vi "Add Mux.vi"(8 "error in (no error)":errorcluster, 11 "Node Ptr":u64 format="%.0x") -> (0 "error out":errorcluster)   [LabVIEW 2013, in "MUX Custom Device.lvlib"]
uses:
  MUX Custom Device.lvlib
  MUX Global.vi
  <vilib>/NI Veristand/Custom Device API/Custom Device API.lvlib
panel:
  in  "Tag":string
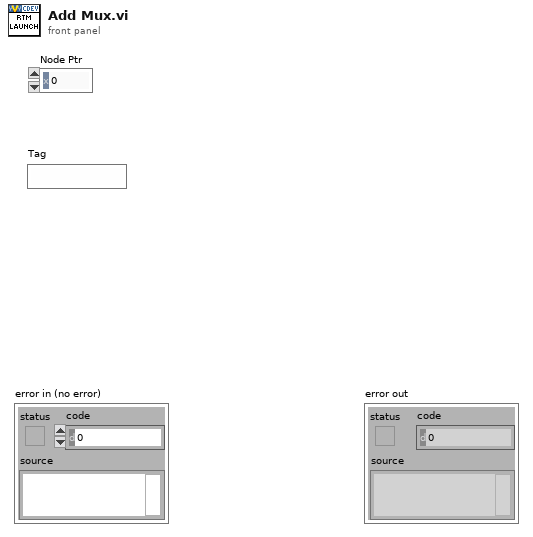
[diagram p1: front panel]
types:
  T1 = typedef "Custom Device API.lvlib/Custom Device Item Ref.ctl" = u64
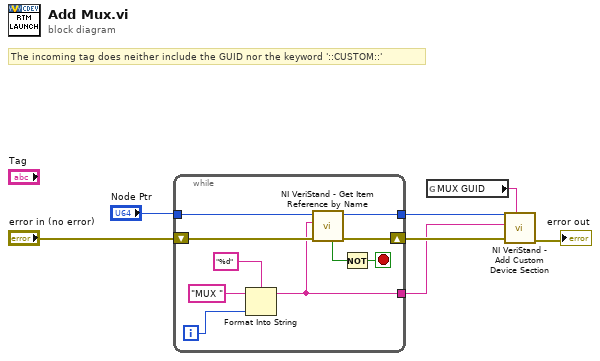
[diagram p0: block diagram]
diagram:
  # "The incoming tag does neither include the GUID nor the keyword '::CUSTOM::'"
  n1 = while {
    tunnel: "Node Ptr" -> [w16]
    shift-right: [w12] -> w2
    shift-left: "error in (no error)" -> [w17]
    tunnel: [w11] -> w3
    tunnel: [w10] -> w1
    i -> [w9]
    stop <- w8 stop-if-true
    n2 = Format Into String(format string="%d", initial string="MUX " ("Label"), w9) -> (resulting string=w10:string)  [unwired: 1 in, 1 out]
    n3 = call <vilib>:"NI VeriStand - Get Item Reference by Name.vi"("error in (no error)"=w17, "Item Name"=w10, "Parent Ref in"=w16) -> ("error out"=w12:errorcluster, "Parent Ref out"=w11:T1, "Found"=w13:bool)  [unwired: 5 in, 1 out]
    n4 = Not(x=w13) -> (.not. x?=w8:bool)
  }
  n5 = global read "MUX Global.vi" "MUX GUID"() -> (w6:string)
  n6 = call <vilib>:"NI VeriStand - Add Custom Device Section.vi"("GUID (Default Section)"=w6, "error in (no error)"=w2, "Section Name"=w1, "Parent Ref in"=w3) -> ("error out"=→"error out":errorcluster)  [unwired: 4 in, 3 out]
